vi "Log State.vi"(8 "error in (no error)":errorcluster, 10 "State":string, 11 "demo in":refnum<class "demo.lvclass">) -> (0 "error out":errorcluster, 3 "demo out":refnum<class "demo.lvclass">)   [LabVIEW 2025, in "demo.lvlib" / "demo.lvclass"]
uses:
  demo.lvclass
  demo.lvclass/demo.ctl
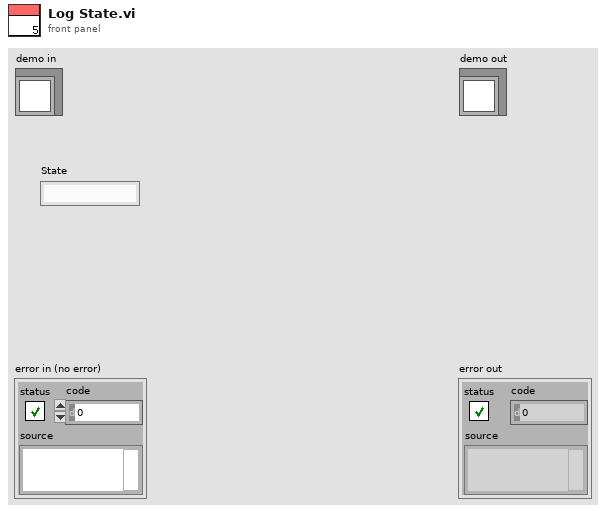
[diagram p1: front panel]
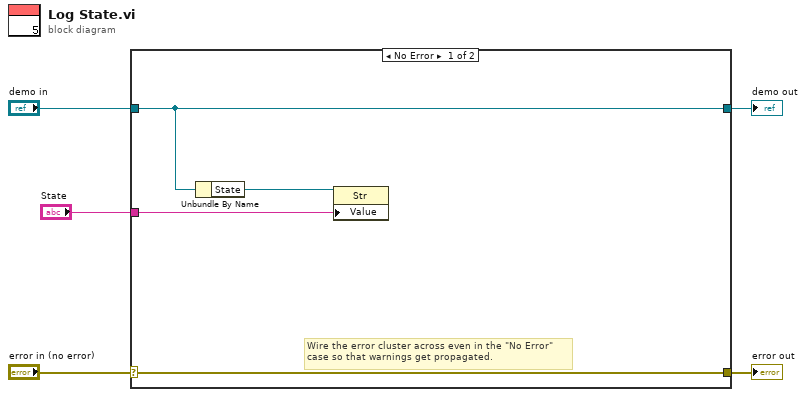
[diagram p0: block diagram]
diagram:
  n1 = case shown="No Error" "error in (no error)" {
    selector: "error in (no error)" -> [w9 w11]
    tunnel: [w9 w11] -> w4
    tunnel: [w8 w10] -> w2
    tunnel: "demo in" -> [w8 w10]
    tunnel: "State" -> [w6 _]
    frame No Error {
      # "Wire the error cluster across even in the \"No Error\"\ncase so that warnings get propagated."
      n2 = Unbundle By Name(w8) -> ("State"=w7:refnum<vi>)
      n3 = property class="Str"(reference=w7, "Value"=w6) -> ()  [unwired: 1 in, 2 out]
    }
    frame Error {
    }
  }
  "error out" <- w4
  "demo out" <- w2
